vi "add mapping.vi"(7 "owner ID":string, 8 "error in":errorcluster, 9 "channel":refnum<class "TBM channel.lvclass">, 10 "tag descriptor":refnum<class "tag descriptor.lvclass">, 11 "engine configuration":refnum<class "engine configuration.lvclass">) -> (0 "error out":errorcluster, 3 "engine configuration out":refnum<class "engine configuration.lvclass">)   [LabVIEW 2013, in "engine configuration.lvclass"]
doc: "This function maps a channel to a tag. A tag can have one writer and multiple readers. Mappings must be made of the same data type."
uses:
  engine configuration.lvclass
  <vilib>/NI/Tag Bus/tag/tag descriptor.lvclass
  <vilib>/NI/Tag Bus Module Framework/channel/TBM channel.lvclass
  <vilib>/NI/Tag Bus/tag/tag descriptor.lvclass/tag descriptor.ctl
  <vilib>/NI/Tag Bus/tag/read tag name.vi
  <vilib>/NI/Tag Bus/tag/read data type.vi
  <vilib>/NI/Configuration Framework/NISE_CEF_TreeControl.lvlib
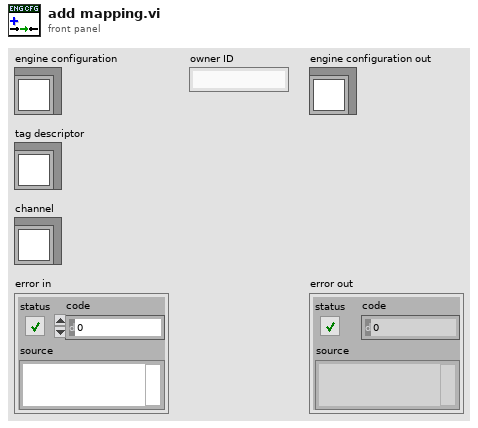
[diagram p1: front panel]
types:
  T1 = typedef "tag bus.lvlib/tag descriptor.lvclass/Data Type.ctl" = enum16{"Double", "Single", "I64", "I32", "I16", "I8", "U64", "U32", "U16", "U8", "Boolean", "String", "Array of Double", "Array of Single", "Array of I64", "Array of I32", "Array of I16", "Array of I8", "Array of U64", "Array of U32", "Array of U16", "Array of U8", "Array of Boolean", "Array of String"}
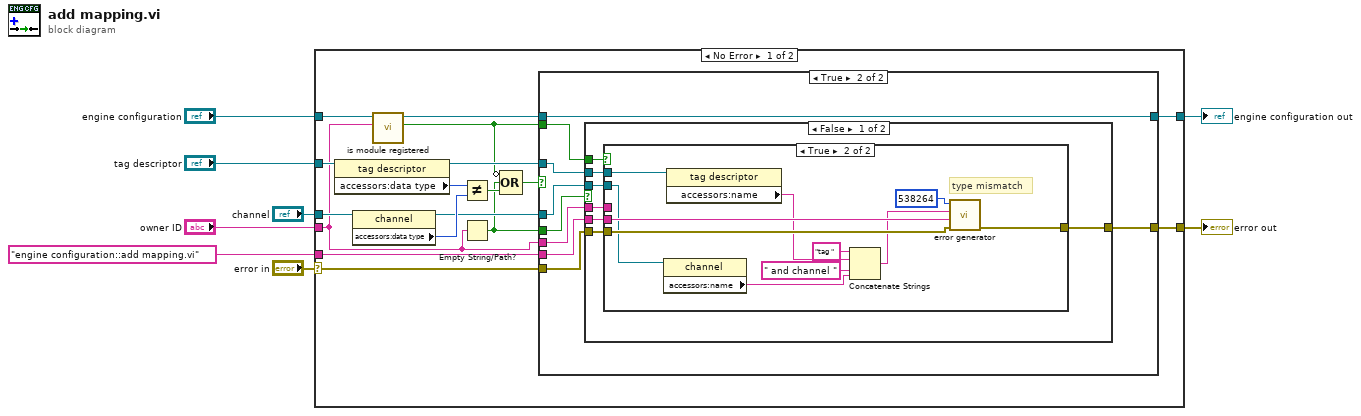
[diagram p0: block diagram]
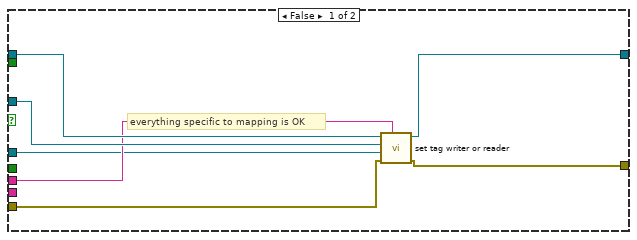
[diagram p2: hidden frame]
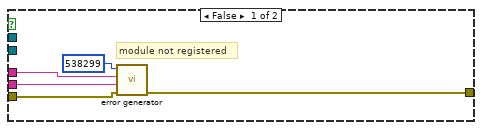
[diagram p3: hidden frame]
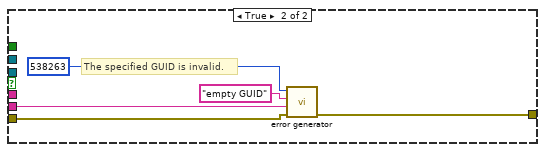
[diagram p4: hidden frame]
diagram:
  n1 = case shown="No Error" "error in" {
    selector: "error in" -> [w20 w70]
    tunnel: "owner ID" -> [w11 _]
    tunnel: "engine configuration" -> [w13 w71]
    tunnel: "tag descriptor" -> [w25 _]
    tunnel: "channel" -> [w24 _]
    tunnel: [w21 w71] -> w4
    tunnel: [w19 w70] -> w2
    tunnel: "engine configuration::add mapping.vi" ("source") -> [w9 _]
    frame No Error {
      n2 = property class="tag descriptor"(reference=w25) -> (reference out=w17:refnum<class "tag descriptor.lvclass">, "accessors:data type"=w22:T1)  [unwired: 1 in, 1 out]
      n3 = property class="channel"(reference=w24) -> (reference out=w18:refnum<class "TBM channel.lvclass">, "accessors:data type"=w23:T1)  [unwired: 1 in, 1 out]
      n4 = call-dynamic "is module registered.vi"("module ID"=w11, "engine configuration in"=w13) -> ("registered?"=w10:bool, "engine configuration out"=w12:refnum<class "engine configuration.lvclass">)  [unwired: 7 in, 1 out]
      n5 = Not Equal?(x=w22, y=w23) -> (x != y?=w16:bool)
      n6 = Empty String/Path?(string/path=w11) -> (empty?=w14:bool)
      n7 = Compound Arithmetic op=OR(invert w10, w14, w16) -> (w15:bool)
      n8 = case shown="True" w15 {
        tunnel: w12 -> [w31 w41]
        tunnel: w11 -> [w29 w36]
        tunnel: [w27 w41] -> w21
        tunnel: w20 -> [w32 w39]
        tunnel: [w26 w38] -> w19
        tunnel: w17 -> [w30 w33]
        tunnel: w18 -> [w28 w34]
        tunnel: w14 -> [_ w40]
        tunnel: w10 -> [_ w37]
        tunnel: w9 -> [_ w35]
        frame False {
          # "everything specific to mapping is OK"
          n9 = call "set tag writer or reader.vi"("module GUID"=w29, "error in"=w32, "channel"=w28, "tag descriptor"=w30, "engine configuration in"=w31) -> ("error out"=w26:errorcluster, "engine configuration out"=w27:refnum<class "engine configuration.lvclass">)  [unwired: 5 in]
        }
        frame True {
          n10 = case shown="False" w40 {
            tunnel: w39 -> [w48 w68]
            tunnel: [w47 w67] -> w38
            tunnel: w37 -> [w46 _]
            tunnel: w36 -> [w45 _]
            tunnel: w35 -> [w44 w66]
            tunnel: w34 -> [w43 _]
            tunnel: w33 -> [w42 _]
            frame False {
              n11 = case shown="True" w46 {
                tunnel: w48 -> [w52 w63]
                tunnel: [w51 w62] -> w47
                tunnel: w45 -> [w50 _]
                tunnel: w44 -> [w49 w61]
                tunnel: w43 -> [_ w59]
                tunnel: w42 -> [_ w60]
                frame False {
                  # "module not registered"
                  n12 = call <vilib>:"error generator.vi"("error in"=w52, "source"=w49, "append error message"=w50, "error code (0)"=538299) -> ("error out"=w51:errorcluster)  [unwired: 5 in]
                }
                frame True {
                  # "type mismatch"
                  n13 = property class="channel"(reference=w59) -> ("accessors:name"=w55:string)  [unwired: 1 in, 2 out]
                  n14 = property class="tag descriptor"(reference=w60) -> ("accessors:name"=w57:string)  [unwired: 1 in, 2 out]
                  n15 = Concatenate Strings("tag " ("string"), w57, " and channel " ("string"), w55) -> (w54:string)
                  n16 = call <vilib>:"error generator.vi"("error in"=w63, "source"=w61, "append error message"=w54, "error code (0)"=538264) -> ("error out"=w62:errorcluster)  [unwired: 5 in]
                }
              }
            }
            frame True {
              # "The specified GUID is invalid."
              n17 = call <vilib>:"error generator.vi"("error in"=w68, "source"=w66, "append error message"="empty GUID", "error code (0)"=538263) -> ("error out"=w67:errorcluster)  [unwired: 5 in]
            }
          }
        }
      }
    }
    frame Error {
    }
  }
  "error out" <- w2
  "engine configuration out" <- w4
